vi "Device Tree Control.vi"() -> ()   [LabVIEW 2013]
panel:
  in  "Device List":string(tree) caption="设备列表"
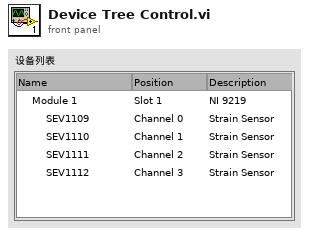
[diagram p1: front panel]
types:
  T1 = cluster{"Left Cell String":string, "Child Text":string[], "Child Tag":string, "Item Indent":i32, "Child Only?":bool, "Glyph Index":i32}[]
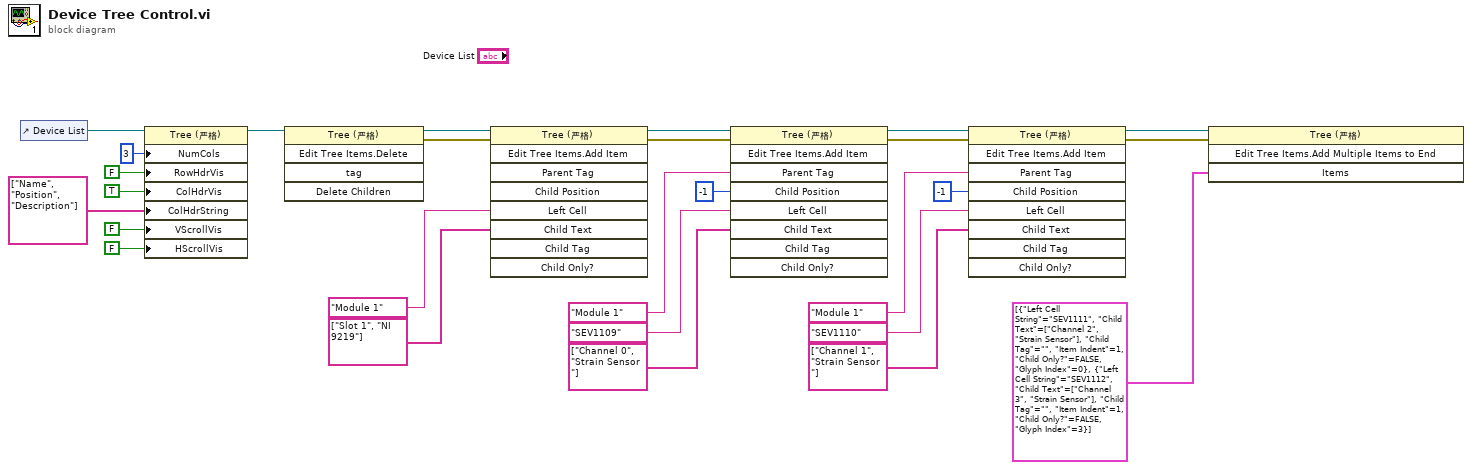
[diagram p0: block diagram]
diagram:
  n1 = control-ref of="Device List"() -> (w27:refnum<vi>)
  n2 = property class="Tree (严格)"(reference=w27, "NumCols"=u32 3 ("列数"), "RowHdrVis"=FALSE ("显示项:显示列首"), "ColHdrVis"=TRUE ("显示项:显示行首"), "ColHdrString"=string[] ["Name", "Position", "Description"], "VScrollVis"=FALSE ("显示项:显示垂直滚动条"), "HScrollVis"=FALSE ("显示项:显示水平滚动条")) -> (reference out=w10:refnum<vi>)  [unwired: 1 in, 1 out]
  n3 = invoke class="Tree (严格)" method="Edit Tree Items.Delete"(reference=w10) -> (reference out=w26:refnum<vi>, error out=w25:errorcluster)  [unwired: 4 in, 3 out]
  n4 = invoke class="Tree (严格)" method="Edit Tree Items.Add Item"(reference=w26, error in=w25, "Left Cell"="Module 1", "Child Text"=string[] ["Slot 1", "NI 9219"]) -> (reference out=w22:refnum<vi>, error out=w21:errorcluster)  [unwired: 5 in, 7 out]
  n5 = invoke class="Tree (严格)" method="Edit Tree Items.Add Item"(reference=w22, error in=w21, "Parent Tag"="Module 1", "Child Position"=-1 ("子项位置"), "Left Cell"="SEV1109", "Child Text"=string[] ["Channel 0", "Strain Sensor "]) -> (reference out=w20:refnum<vi>, error out=w19:errorcluster)  [unwired: 3 in, 7 out]
  n6 = invoke class="Tree (严格)" method="Edit Tree Items.Add Item"(reference=w20, error in=w19, "Parent Tag"="Module 1", "Child Position"=-1 ("子项位置"), "Left Cell"="SEV1110", "Child Text"=string[] ["Channel 1", "Strain Sensor "]) -> (reference out=w9:refnum<vi>, error out=w8:errorcluster)  [unwired: 3 in, 7 out]
  n7 = invoke class="Tree (严格)" method="Edit Tree Items.Add Multiple Items to End"(reference=w9, error in=w8, "Items"=T1 [{"Left Cell String"="SEV1111", "Child Text"=["Channel 2", "Strain Sensor"], "Child Tag"="", "Item Indent"=1, "Child Only?"=FALSE, "Glyph Index"=0}, {"Left Cell String"="SEV1112", "Child Text"=["Channel 3", "Strain Sensor"], "Child Tag"="", "Item Indent"=1, "Child Only?"=FALSE, "Glyph Index"=3}] ("多项")) -> ()  [unwired: 1 in, 4 out]
